vi "Prueba1.vi"() -> ()   [LabVIEW 2020]
uses:
  <vilib>/Utility/config.llb/Read Key (Double).vi
  <vilib>/Utility/config.llb/Read Key (String).vi
  <vilib>/Utility/config.llb/NI_LVConfig.lvlib
panel:
  out "element 3":string
  out "element 2":string
  out "element":string
  out "subarray":string[](array[string])
  in  "s":bool
  out "Numeric":dbl
  in  "stop":bool
  in  "Productos":i32(listbox)
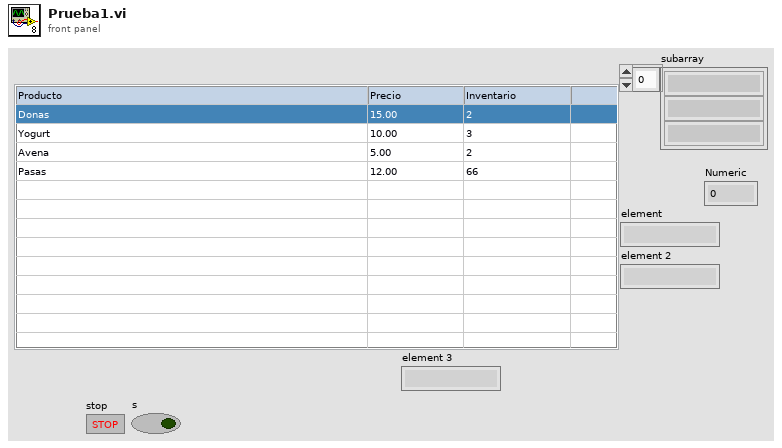
[diagram p1: front panel]
types:
  T1 = typedef "NI_LVConfig.lvlib/Config Data RefNum.ctl" = refnum<k1>
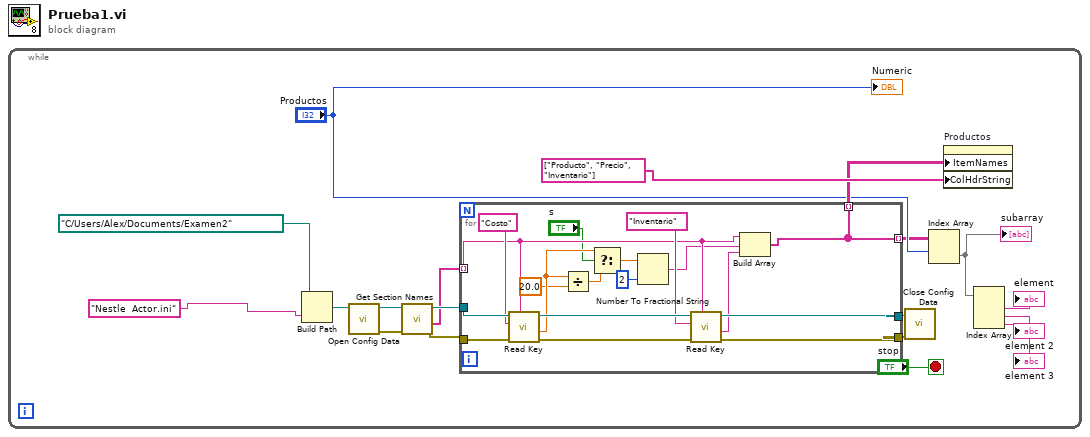
[diagram p0: block diagram]
diagram:
  n1 = while {
    stop <- "stop" stop-if-true
    n2 = Build Path(base path=path "C:/Users/Alex/Documents/Examen2", name or relative path="Nestle  Actor.ini" ("string")) -> (appended path=w18:path)
    n3 = call <vilib>:"Open Config Data.vi"("configuration file path"=w18) -> ("error out"=w14:errorcluster, "refnum"=w15:T1)  [unwired: 8 in, 1 out]
    n4 = call <vilib>:"Get Section Names.vi"("error in (no error)"=w14, "refnum"=w15) -> ("error out"=w12:errorcluster, "section names"=w11:string[], "refnum out"=w13:T1)  [unwired: 7 in]
    n5 = for {
      tunnel: w13 -> [w37]
      tunnel: [w34] -> w17
      tunnel: [w33] -> w16
      tunnel: w12 -> [w30]
      tunnel: w11 -> [w27] mode=indexing
      tunnel: [w20] -> w7 mode=indexing
      tunnel: [w20] -> w5 mode=indexing
      n6 = call-poly <vilib>:"Read Key.vi"("section"=w27, "error in (no error)"=w30, "key"="Costo", "refnum"=w37) -> ("error out"=w36:errorcluster, "value"=w23:dbl, "refnum out"=w35:T1)  [unwired: 4 in, 1 out]
      n7 = Divide(x=w23, y=20.0) -> (x/y=w24:dbl)
      n8 = Select(t=w23, s="s", f=w24) -> (s? t:f=w25:dbl)
      n9 = Number To Fractional String(number=w25, precision (6)=i16 2) -> (F-format string=w26:string)  [unwired: 2 in]
      n10 = call-poly <vilib>:"Read Key.vi"("section"=w27, "error in (no error)"=w36, "key"="Inventario", "refnum"=w35) -> ("error out"=w33:errorcluster, "value"=w28:string, "refnum out"=w34:T1)  [unwired: 4 in, 1 out]
      n11 = Build Array(w27, w26, w28) -> (w20:string[])
    }
    n12 = call <vilib>:"Close Config Data.vi"("error in (no error)"=w16, "refnum"=w17) -> ()  [unwired: 8 in, 2 out]
    n13 = Index Array(array=w5, index (row)="Productos") -> (element=w4:string[])  [unwired: 1 in]
    "subarray" <- w4
    n14 = property on="Productos" class="MCListbox (strict)"("ItemNames"=w7, "ColHdrString"=string[] ["Producto", "Precio", "Inventario"] ("Column Header Strings[]")) -> ()  [unwired: 2 in, 2 out]
    n15 = Index Array(array=w4) -> (element #1=→"element":string, element #2=→"element 2":string, element #3=→"element 3":string)  [unwired: 3 in]
    "Numeric" <- "Productos"
  }
